vi "Match tag img.vi"(7 "String":string, 11 "error in (no error)":errorcluster) -> (4 "Position [ ]":i32[](array[numeric]), 8 "Text [ ]":cluster{"String":string, "Image?":bool}[](array[cluster]), 15 "error out":errorcluster)   [LabVIEW 2012]
doc: "Version 1.0\nDeveloped by Jean-Marc Simard\nCopyright © 2010, Exaprom Inc.\nAll rights reserved.\nLicense: BSD"
panel:
  out "x-y":u32
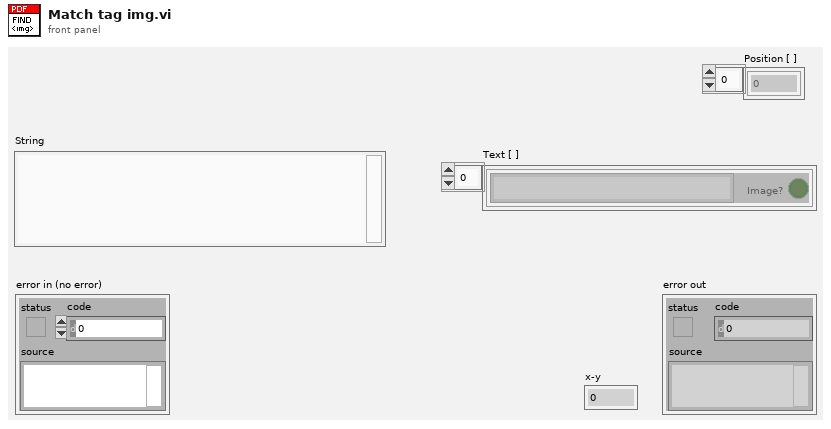
[diagram p1: front panel]
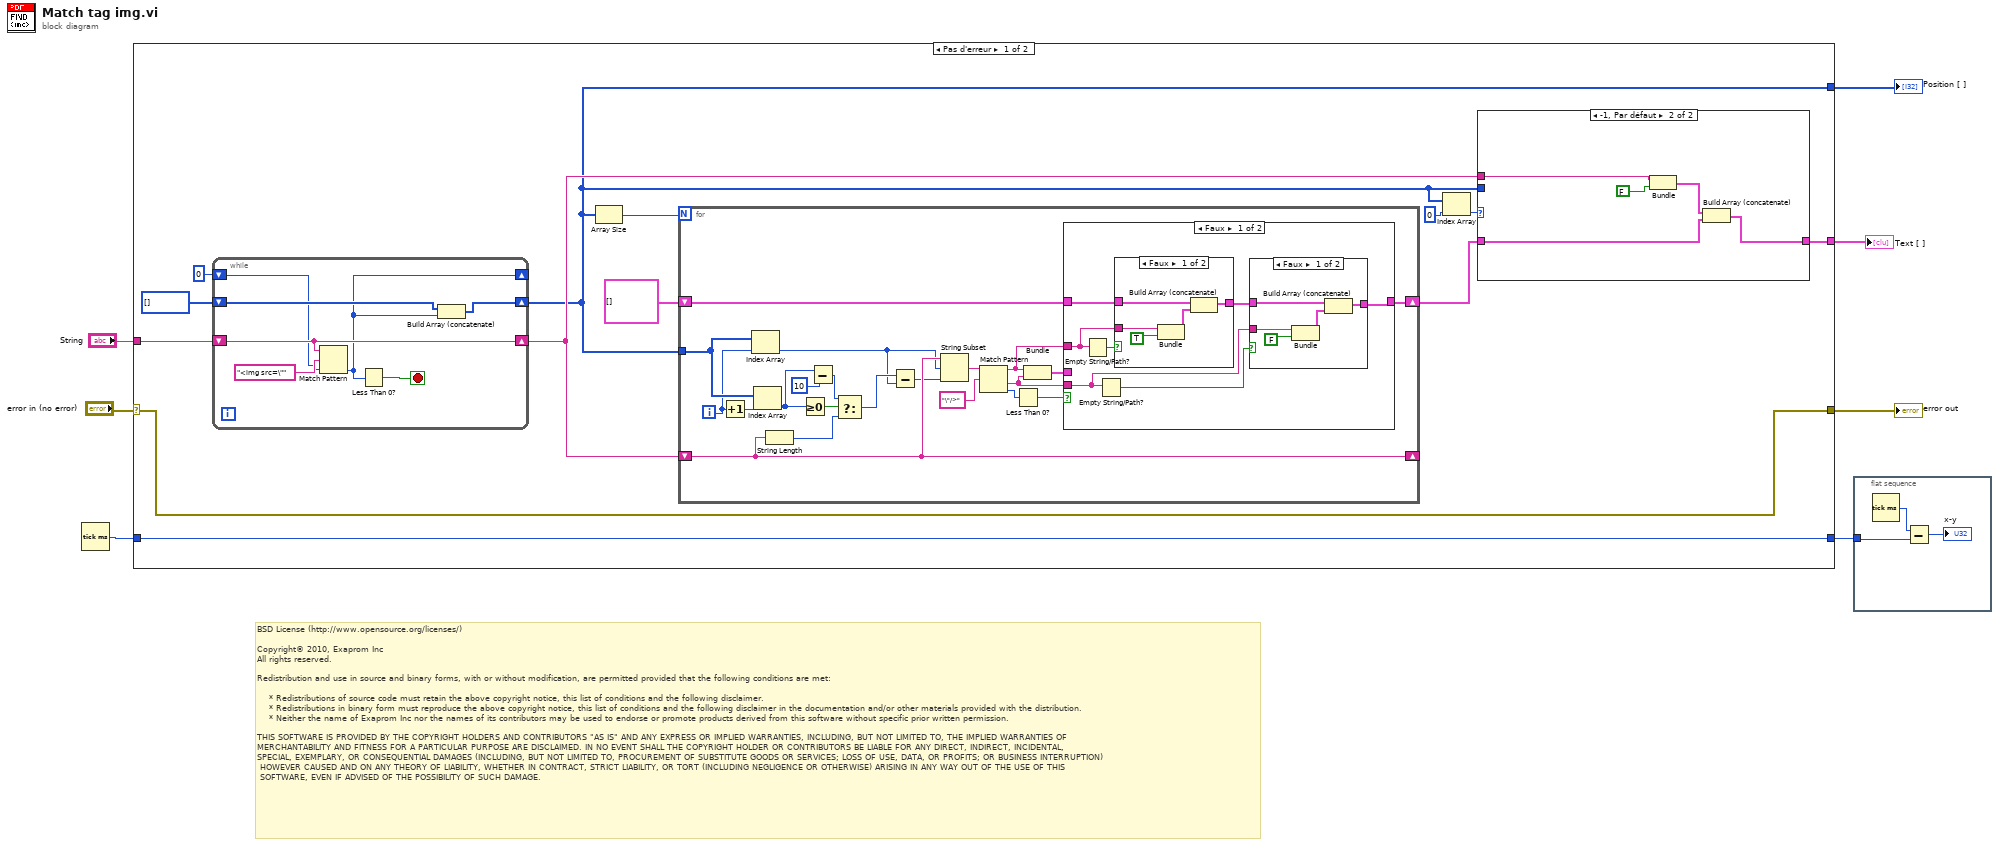
[diagram p0: block diagram]
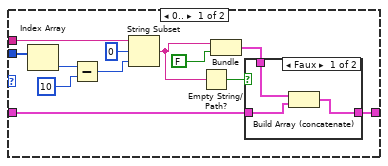
[diagram p5: hidden frame]
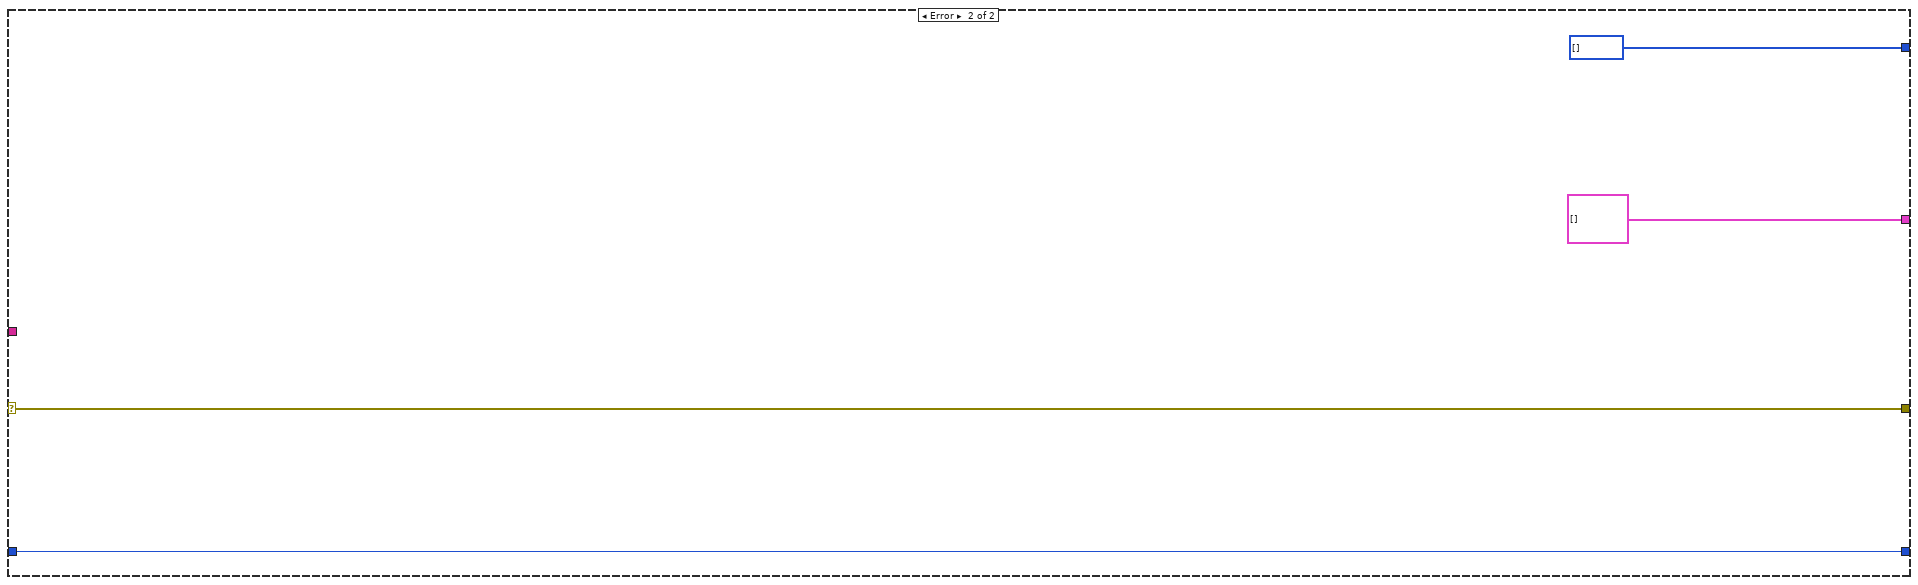
[diagram p7: hidden frame]
diagram:
  # "BSD License (http://www.opensource.org/licenses/)\n\nCopyright© 2010, Exaprom Inc\nAll rights reserved.\n\nRedistribution and use in source and binary forms, with or without modification, are permitted provided that the following conditions are met:\n\n    * Redistributions of source code must retain the above copyright notice, this list of conditions and the following disclaimer.\n    * Redistributions in binary form must reproduce the above copyright notice, this list of conditions and the following disclaimer in the documentation and/or other materials provided with the distribution.\n    * Neither the name of Exaprom Inc nor the names of its contributors may be used to endorse or promote products derived from this software without specific prior written permission.\n\nTHIS SOFTWARE IS PROVIDED BY THE COPYRIGHT HOLDERS AND CONTRIBUTORS \"AS IS\" AND ANY EXPRESS OR IMPLIED WARRANTIES, INCLUDING, BUT NOT LIMITED TO, THE IMPLIED WARRANTIES OF \nMERCHANTABILITY AND FITNESS FOR A PARTICULAR PURPOSE ARE DISCLAIMED. IN NO EVENT SHALL THE COPYRIGHT HOLDER OR CONTRIBUTORS BE LIABLE FOR ANY DIRECT, INDIRECT, INCIDENTAL,\nSPECIAL, EXEMPLARY, OR CONSEQUENTIAL DAMAGES (INCLUDING, BUT NOT LIMITED TO, PROCUREMENT OF SUBSTITUTE GOODS OR SERVICES; LOSS OF USE, DATA, OR PROFITS; OR BUSINESS INTERRUPTION)\n HOWEVER CAUSED AND ON ANY THEORY OF LIABILITY, WHETHER IN CONTRACT, STRICT LIABILITY, OR TORT (INCLUDING NEGLIGENCE OR OTHERWISE) ARISING IN ANY WAY OUT OF THE USE OF THIS\n SOFTWARE, EVEN IF ADVISED OF THE POSSIBILITY OF SUCH DAMAGE."
  n1 = Tick Count (ms)() -> (millisecond timer value=w2:u32)
  n2 = case shown="Pas d'erreur" "error in (no error)" {
    selector: "error in (no error)" -> [w9 w93]
    tunnel: "String" -> [w18 _]
    tunnel: [w12 cluster{"String":string, "Image?":bool}[] [] ("Text [ ]")] -> w3
    tunnel: [w9 w93] -> w6
    tunnel: [w11 i32[] []] -> w4
    tunnel: w2 -> [w8 w90]
    tunnel: [w8 w90] -> w1
    frame No Error {
      n3 = while {
        shift-right: [w64] -> w16
        shift-left: w18 -> [w64]
        shift-right: [w67] -> w11
        shift-left: i32[] [] -> [w66]
        shift-right: [w63] -> _
        shift-left: 0 -> [w62]
        stop <- w65 stop-if-true
        n4 = Match Pattern(string=w64, regular expression="<img src=\"", offset (0)=w62) -> (offset past match=w63:i32)  [unwired: 3 out]
        n5 = Less Than 0?(x=w63) -> (x < 0?=w65:bool)
        n6 = Build Array (concatenate)(w66, w63) -> (w67:i32[])
      }
      n7 = Array Size(array=w11) -> (size(s)=w19:i32)
      n8 = for {
        N: w19 -> [_]
        shift-right: [w37] -> _
        shift-left: w16 -> [w37]
        tunnel: w11 -> [w41]
        shift-right: [w24] -> w13
        shift-left: cluster{"String":string, "Image?":bool}[] [] ("Text [ ]") -> [w25]
        i -> [w40]
        n9 = Increment(x=w40) -> (x+1=w39:i32)
        n10 = Index Array(array=w41, index=w40) -> (element=w32:i32)
        n11 = Index Array(array=w41, index=w39) -> (element=w36:i32)
        n12 = String Length(string=w37) -> (length=w28:i32)
        n13 = Greater Or Equal To 0?(x=w36) -> (x >= 0?=w38:bool)
        n14 = Subtract(x=w36, y=10) -> (x-y=w34:i32)
        n15 = Select(t=w34, s=w38, f=w28) -> (s? t:f=w33:i32)
        n16 = Subtract(x=w33, y=w32) -> (x-y=w31:i32)
        n17 = String Subset(string=w37, offset (0)=w32, length (rest)=w31) -> (substring=w29:string)
        n18 = Match Pattern(string=w29, regular expression="\"/>") -> (before substring=w22:string, after substring=w21:string, offset past match=w27:i32)  [unwired: 2 out]
        n19 = Less Than 0?(x=w27) -> (x < 0?=w26:bool)
        n20 = Bundle("String"=w22, "String"=w21) -> (w23:cluster{"String":string, "String":string})  [unwired: 1 out]
        n21 = case shown="Faux" w26 {
          tunnel: w25 -> [w46 w61]
          tunnel: [w45 w61] -> w24
          tunnel: w23 -> [_ _]
          tunnel: w22 -> [w47 _]
          tunnel: w21 -> [w42 _]
          frame False {
            n22 = Empty String/Path?(string/path=w47) -> (empty?=w48:bool)
            n23 = Empty String/Path?(string/path=w42) -> (empty?=w43:bool)
            n24 = case shown="Faux" w48 {
              tunnel: w47 -> [w57 _]
              tunnel: [w59 w60] -> w44
              tunnel: w46 -> [w58 w60]
              frame False {
                n25 = Bundle("String"=w57, TRUE) -> (w56:cluster{"String":string, bool})  [unwired: 1 out]
                n26 = Build Array (concatenate)(w58, w56) -> (w59:cluster{"String":string, "Image?":bool}[])
              }
              frame True {
              }
            }
            n27 = case shown="Faux" w43 {
              tunnel: w42 -> [w51 _]
              tunnel: [w53 w54] -> w45
              tunnel: w44 -> [w52 w54]
              frame False {
                n28 = Bundle("String"=w51, FALSE) -> (w50:cluster{"String":string, bool})  [unwired: 1 out]
                n29 = Build Array (concatenate)(w52, w50) -> (w53:cluster{"String":string, "Image?":bool}[])
              }
              frame True {
              }
            }
          }
          frame True {
          }
        }
      }
      n30 = Index Array(array=w11, index=0) -> (element=w15:i32)
      n31 = case shown="-1, Par défaut" w15 {
        tunnel: w16 -> [w80 w86]
        tunnel: w11 -> [w75 _]
        tunnel: w13 -> [w74 w89]
        tunnel: [w72 w87] -> w12
        frame 0.. {
          n32 = Index Array(array=w75) -> (element=w78:i32)  [unwired: 1 in]
          n33 = Subtract(x=w78, y=10) -> (x-y=w76:i32)
          n34 = String Subset(string=w80, offset (0)=0, length (rest)=w76) -> (substring=w70:string)
          n35 = Empty String/Path?(string/path=w70) -> (empty?=w71:bool)
          n36 = Bundle("String"=w70, FALSE) -> (w73:cluster{"String":string, bool})  [unwired: 1 out]
          n37 = case shown="Faux" w71 {
            tunnel: w74 -> [w83 w84]
            tunnel: w73 -> [w82 _]
            tunnel: [w81 w84] -> w72
            frame False {
              n38 = Build Array (concatenate)(w82, w83) -> (w81:cluster{"String":string, "Image?":bool}[])
            }
            frame True {
            }
          }
        }
        frame -1, Default {
          n39 = Bundle("String"=w86, FALSE) -> (w88:cluster{"String":string, bool})  [unwired: 1 out]
          n40 = Build Array (concatenate)(w88, w89) -> (w87:cluster{"String":string, "Image?":bool}[])
        }
      }
    }
    frame Error {
    }
  }
  "error out" <- w6
  "Position [ ]" <- w4
  "Text [ ]" <- w3
  n41 = flat-sequence {
    tunnel: w1 -> [w95]
    frame #0 {
      n42 = Tick Count (ms)() -> (millisecond timer value=w96:u32)
      n43 = Subtract(x=w96, y=w95) -> (x-y=→"x-y":u32)
    }
  }
